vi "CHD_ODOM_EXECUTE.vi"(6 "Pass_Through_Time":dbl=-1.0 format="%33.4f", 8 "error in (no error)":errorcluster) -> (0 "error out":errorcluster)   [LabVIEW 2019]
uses:
  <vilib>/Rock Robotics/WPI/ThirdParty/JAS_Junk/TrajLib/Rotation2d_Minus.vi
  <vilib>/Rock Robotics/WPI/ThirdParty/JAS_Junk/TrajLib/Rotation2d_Plus.vi
  <vilib>/Rock Robotics/WPI/ThirdParty/JAS_Junk/TrajLib/Twist2d_Create.vi
  <vilib>/Rock Robotics/WPI/ThirdParty/JAS_Junk/TrajLib/Rotation2d_GetRadians.vi
  <vilib>/Rock Robotics/WPI/ThirdParty/JAS_Junk/TrajLib/VI/Util_GetTime_U32.vi
  <vilib>/Rock Robotics/WPI/ThirdParty/JAS_Junk/TrajLib/Rotation2d_UnaryMinus.vi
  <vilib>/Rock Robotics/WPI/ThirdParty/JAS_Junk/TrajLib/Rotation2d_RotateBy.vi
  <vilib>/Rock Robotics/WPI/ThirdParty/JAS_Junk/TrajLib/Rotation2d_CreateXY.vi
  <vilib>/Rock Robotics/WPI/ThirdParty/JAS_Junk/TrajLib/Util_CalcDist.vi
  Differential_Drive_System/CHD_DRIVE_GLOBALS.vi
  CHD_ODOM_GLOBALS.vi
  <vilib>/Rock Robotics/WPI/ThirdParty/JAS_Junk/TrajLib/Pose2d_Exp.vi
  <vilib>/Rock Robotics/WPI/ThirdParty/JAS_Junk/TrajLib/VI/Util_GetTime_U64.vi
  <vilib>/Rock Robotics/WPI/ThirdParty/JAS_Junk/TrajLib/Trajectory_Library.lvlib
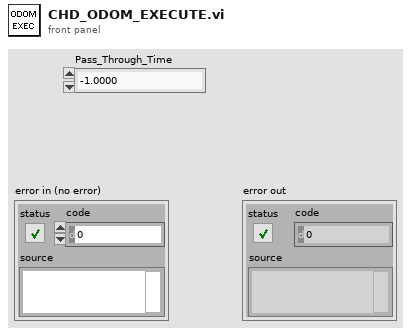
[diagram p1: front panel]
types:
  T1 = typedef "Trajectory_Library.lvlib/DIFF_DRIVE_ODOM2.ctl" = cluster{"M_POSE_Meters":T2, "M_GyroOffset":T4, "M_PrevAngle":T4, "M_PrevLeftDist_M":dbl, "M_PrevRightDist_M":dbl, "M_InitLeftDist_M":dbl, "M_InitRightDist_M":dbl}
  T2 = typedef "Trajectory_Library.lvlib/POSE2D.ctl" = cluster{"TRANSLATION":T3, "ROTATION":T4}
  T3 = typedef "Trajectory_Library.lvlib/TRANSLATION2D.ctl" = cluster{"X":dbl, "Y":dbl}
  T4 = typedef "Trajectory_Library.lvlib/ROTATION2D.ctl" = cluster{"VALUE":dbl, "COS":dbl, "SIN":dbl}
  T5 = typedef "Trajectory_Library.lvlib/DIFF_DRIVE_KINEMATICS.ctl" = cluster{"TrackWidth_Meters":dbl}
  T6 = typedef "Trajectory_Library.lvlib/DIFF_DRIVE_POSE_EST2_CONFIG.ctl" = cluster{"TrackWidth_Meters":dbl, "Odom X std dev M":dbl, "Odom Y std dev M":dbl, "Odom Heading std dev Rad":dbl, "Vision X std dev M":dbl, "Vision Y std dev M":dbl, "Vision Heading std dev Rad":dbl}
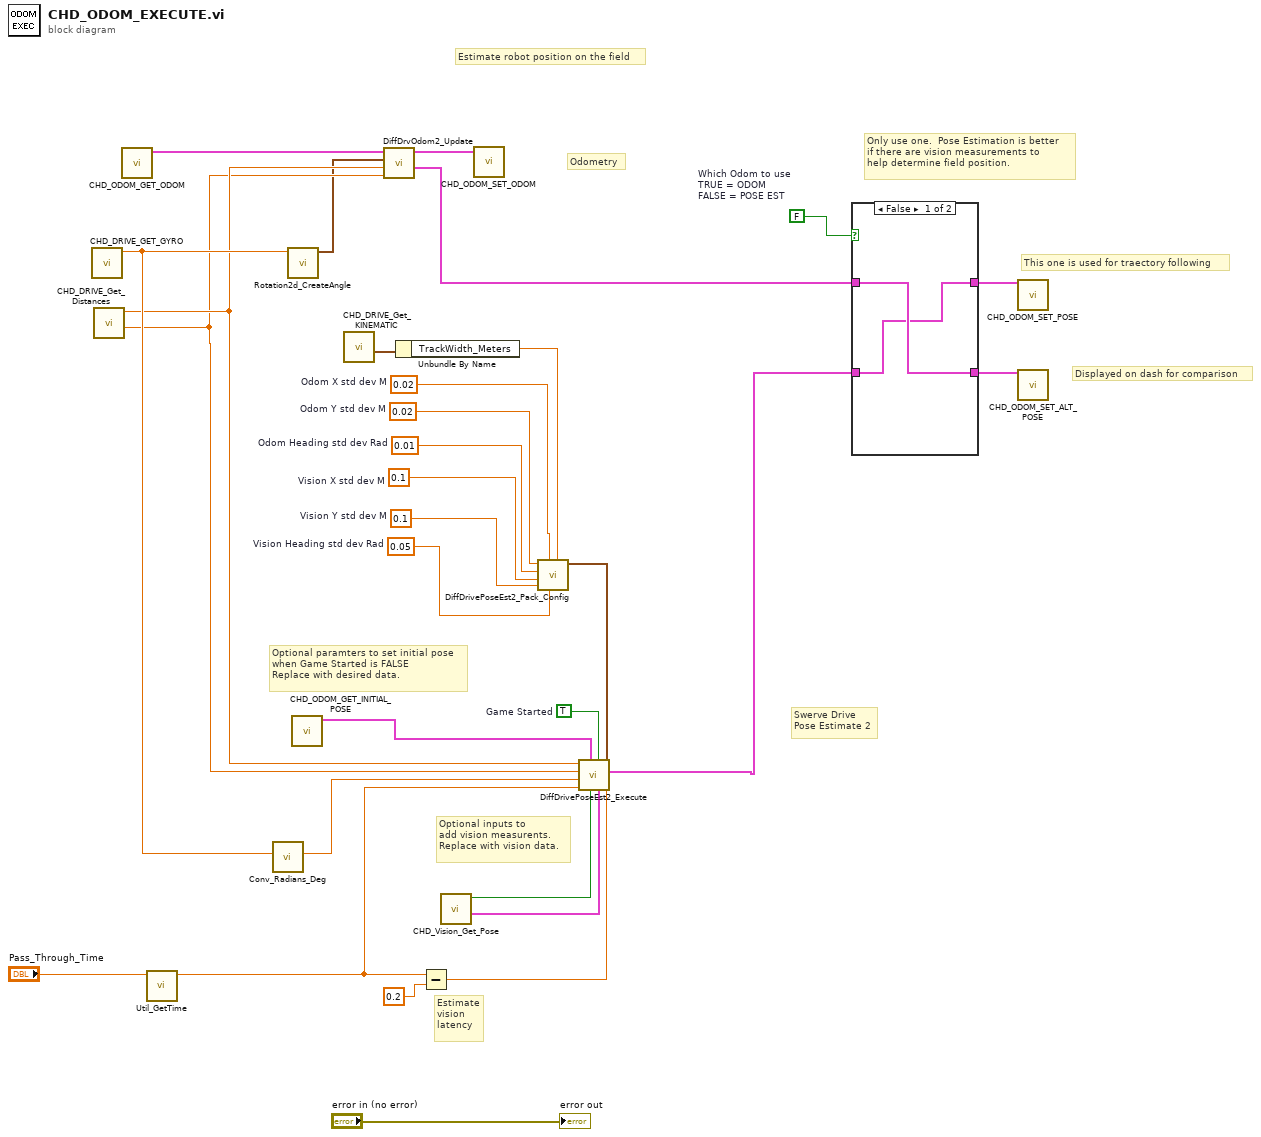
[diagram p0: block diagram]
diagram:
  w5 = 0.02  # Odom Y std dev M
  w6 = 0.01  # Odom Heading std dev Rad
  w7 = 0.1  # Vision X std dev M
  w8 = 0.1  # Vision Y std dev M
  w9 = 0.02  # Odom X std dev M
  w10 = 0.05  # Vision Heading std dev Rad
  w26 = FALSE  # Which Odom to use TRUE = ODOM FALSE = POSE EST
  w24 = TRUE  # Game Started
  # "Displayed on dash for comparison"
  # "Estimate\nvision \nlatency"
  # "This one is used for traectory following"
  # "Only use one.  Pose Estimation is better\nif there are vision measurements to\nhelp determine field position."
  # "Optional inputs to\nadd vision measurents.\nReplace with vision data."
  # "Optional paramters to set initial pose\nwhen Game Started is FALSE\nReplace with desired data."
  # "Swerve Drive \nPose Estimate 2"
  # "Odometry"
  # "Estimate robot position on the field"
  n1 = call "CHD_DRIVE_GET_GYRO.vi"() -> ("Gyro Heading Radians"=w28:dbl)  [unwired: 11 in]
  n2 = call "CHD_DRIVE_Get_Distances.vi"() -> ("RightDistance_M"=w22:dbl, "LeftDistance_M"=w23:dbl)  [unwired: 9 in, 1 out]
  n3 = call "CHD_ODOM_GET_ODOM.vi"() -> ("Absolue Odometry"=w12:T1)  [unwired: 11 in]
  n4 = call <vilib>:"Util_GetTime.vi"("Pass_Through_Time"="Pass_Through_Time") -> ("FPGA_Time_Seconds"=w19:dbl)  [unwired: 8 in, 2 out]
  n5 = call <vilib>:"Conv_Radians_Deg.vi"("Radians"=w28) -> ("Degrees"=w20:dbl)  [unwired: 10 in]
  n6 = call <vilib>:"Rotation2d_CreateAngle.vi"("Angle"=w28) -> ("ROTATION"=w14:T4)  [unwired: 10 in]
  n7 = call "CHD_ODOM_GET_INITIAL_POSE.vi"() -> ("Initial Odometry Pose"=w2:T2)  [unwired: 11 in]
  n8 = call "CHD_DRIVE_Get_KINEMATIC.vi"() -> ("out DIFF_DRIVE_KINEMATICS"=w4:T5)  [unwired: 11 in]
  n9 = call <vilib>:"DiffDrvOdom2_Update.vi"("Right Distance M"=w22, "Left Distance M"=w23, "Gyro Reading"=w14, "In DIFF_DRIVE_ODOM"=w12) -> ("Pose Meters"=w13:T2, "Out DIFF_DRIVE_ODOM"=w11:T1)  [unwired: 6 in]
  n10 = Unbundle By Name(w4) -> ("TrackWidth_Meters"=w3:dbl)
  n11 = Subtract(x=w19, y=0.2) -> (x-y=w17:dbl)
  n12 = call "CHD_Vision_Get_Pose.vi"() -> ("Vison Pose"=w18:T2, "Have Vision Pose"=w16:bool)  [unwired: 10 in]
  n13 = call "CHD_ODOM_SET_ODOM.vi"("Absolue Odometry"=w11) -> ()  [unwired: 11 in]
  n14 = call <vilib>:"DiffDrivePoseEst2_Pack_Config.vi"("TrackWidth_Meters"=w3, "Vision Heading std dev Rad"=w10, "Odom X std dev M"=w9, "Vision Y std dev M"=w8, "Vision X std dev M"=w7, "Odom Heading std dev Rad"=w6, "Odom Y std dev M"=w5) -> ("DiffPoseEst2Config"=w21:T6)  [unwired: 4 in]
  n15 = call <vilib>:"DiffDrivePoseEst2_Execute.vi"("Vision TImeStamp_Seconds"=w17, "DiffPoseEst2Config"=w21, "visionRobotPose"=w18, "Game Started"=w24, "Add Vision Meas"=w16, "InitialPose"=w2, "Pass Through Time"=w19, "Gyro Degrees"=w20, "RightDistance_M"=w22, "LeftDistance_M"=w23) -> ("Estimated Pose"=w15:T2)  [unwired: 1 out]
  n16 = case shown="False" w26 {
    tunnel: w13 -> [w32 w34]
    tunnel: [w31 w34] -> w27
    tunnel: w15 -> [w31 w33]
    tunnel: [w32 w33] -> w1
    frame False {
    }
    frame True {
    }
  }
  n17 = call "CHD_ODOM_SET_POSE.vi"("Absolute Odometry Pose"=w27) -> ()  [unwired: 11 in]
  n18 = call "CHD_ODOM_SET_ALT_POSE.vi"("Odometry ALT Pose"=w1) -> ()  [unwired: 11 in]
  "error out" <- "error in (no error)"
